vi "rad_Blacklist Help.vi"() -> ()   [LabVIEW 2013]
uses:
  Util/FP Control/FP Control Functions.ctl
panel:
  in  "OK":bool
  # "The Retrieve Blacklist specifies the list of files and folders to exclude when retrieving an image.  This feature can be used to reduce the size of the resulting image. \n\nThe Deploy Blacklist specifies the list of files and folders to protect on the target during a deployment. Files in the blacklist will not be modified on the target during a deployment, even if those files are also contained in the deployment image.  This feature can be used to persist data or configuration files on the target during software updates.\n\nDeployment Blacklist Example\nFor this example, consider the following scenario:\n\nThe image contains files A, B,C, D. \nThe target contains files A, B, E, F. \nThe user blacklist contains files A, C, E, G. \n\nResults:\nFile A on the target is not modified despite being in the image because it is in the blacklist. \nFile B from the image is written over the one on the target. \nFile C from the image is not written to the target because it is in the blacklist. \nFile D from the image is written to the target. \nFile E on the target is not part of the image but is not deleted because it is in the blacklist. \nFile F on the target gets deleted because it is not part of the image. \nFile G in the blacklist is ignored because it is part of neither the image nor the target."
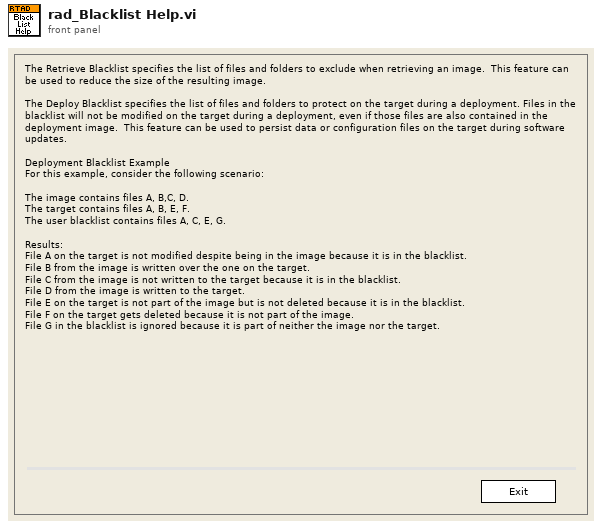
[diagram p1: front panel]
types:
  T1 = typedef "FP Control Functions.ctl" = enum16{"Open", "Close", "Bring To Front", "Center"}
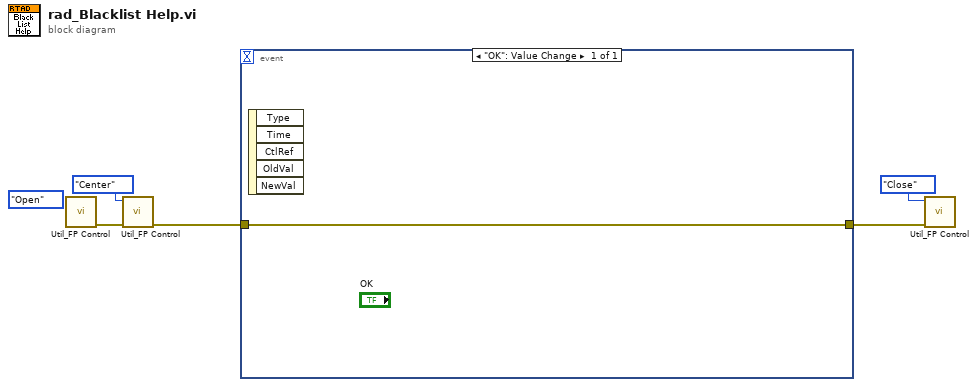
[diagram p0: block diagram]
diagram:
  (unwired) FP_Control_Functions."Open" ("Function")
  n1 = call "Util_FP Control.vi"() -> ("error out"=w4:errorcluster)  [unwired: 2 in, 9 out]
  n2 = call "Util_FP Control.vi"("error in (no error)"=w4, "Function"=FP_Control_Functions."Center") -> ("error out"=w3:errorcluster)  [unwired: 9 out]
  n3 = event shown="[0] \"OK\": Value Change" {
    selector: _ -> [_]
    dyn-events: _ -> [_]
    timeout: _ -> [_]
    tunnel: w3 -> [w6]
    tunnel: [w6] -> w2
    event "OK": Value Change {
      n4 = event-data() -> ()  [unwired: 1 in, 5 out]
    }
  }
  n5 = call "Util_FP Control.vi"("error in (no error)"=w2, "Function"=FP_Control_Functions."Close") -> ()  [unwired: 10 out]
